vi "Binding Machine.vi"() -> ()   [LabVIEW 2014]
uses:
  Master/Master.lvclass
panel:
  in  "Enter":bool
  in  "stop":bool
  out "error out":errorcluster
  in  "error in":errorcluster
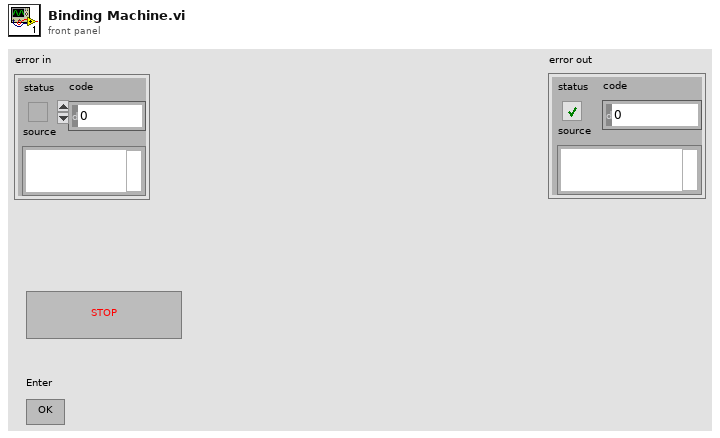
[diagram p1: front panel]
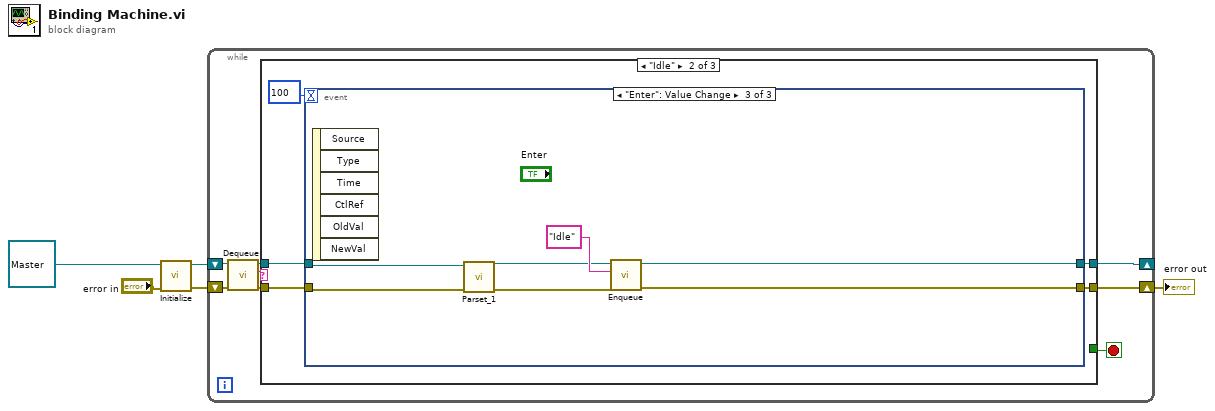
[diagram p0: block diagram]
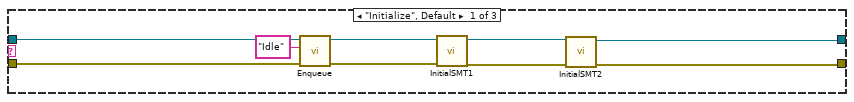
[diagram p2: hidden frame]
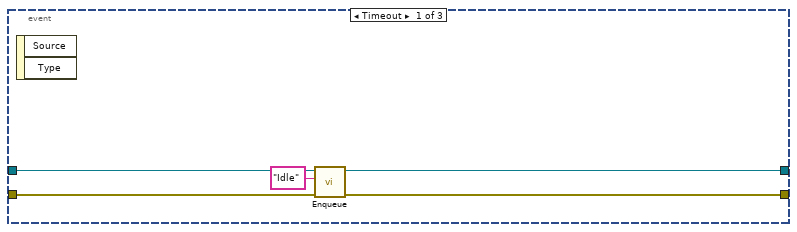
[diagram p3: hidden frame]
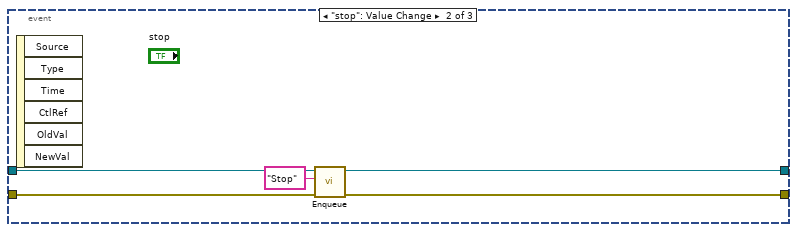
[diagram p4: hidden frame]
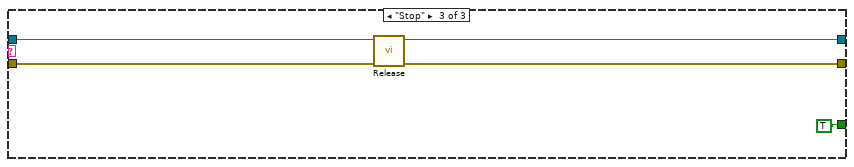
[diagram p5: hidden frame]
diagram:
  n1 = call-dynamic "Initialize.vi"("error in (no error)"="error in", "Master in"=refnum<class "Master.lvclass"> refnum ("Master.lvclass")) -> ("error out"=w2:errorcluster, "Master out"=w3:refnum<class "Master.lvclass">)  [unwired: 8 in]
  n2 = while {
    shift-right: [w9] -> _
    shift-left: w3 -> [w13]
    shift-right: [w7] -> w5
    shift-left: w2 -> [w12]
    stop <- w6 stop-if-true
    n3 = call-dynamic "Dequeue.vi"("error in (no error)"=w12, "Master in"=w13) -> ("error out"=w8:errorcluster, "State"=w11:string, "Master out"=w10:refnum<class "Master.lvclass">)  [unwired: 7 in]
    n4 = case shown="\"Idle\"" w11 {
      tunnel: w10 -> [w20 w26 w48]
      tunnel: [w16 w23 w46] -> w9
      tunnel: w8 -> [w22 w25 w47]
      tunnel: [w14 w24 w45] -> w7
      tunnel: [_ _ TRUE] -> w6
      frame "Initialize", Default {
        n5 = call-dynamic "Enqueue.vi"("error in (no error)"=w22, "State"="Idle", "Master in"=w20) -> ("error out"=w18:errorcluster, "Master out"=w19:refnum<class "Master.lvclass">)  [unwired: 7 in]
        n6 = call-dynamic "InitialSMT1.vi"("error in (no error)"=w18, "Programing Logic in"=w19) -> ("error out"=w15:errorcluster, "Programing Logic out"=w17:refnum<class "Master.lvclass">)  [unwired: 8 in]
        n7 = call-dynamic "InitialSMT2.vi"("error in (no error)"=w15, "Programing Logic in"=w17) -> ("error out"=w14:errorcluster, "Programing Logic out"=w16:refnum<class "Master.lvclass">)  [unwired: 8 in]
      }
      frame "Idle" {
        n8 = event shown="[2] \"Enter\": Value Change" {
          selector: _ -> [_ _ _]
          dyn-events: _ -> [_ _ _]
          timeout: 100 -> [_ _ _]
          tunnel: w26 -> [w32 w37 w43]
          tunnel: w25 -> [w31 w36 w42]
          tunnel: [w30 w35 w39] -> w24
          tunnel: [w29 w34 w38] -> w23
          event Timeout {
            n9 = event-data() -> ()  [unwired: 1 in, 2 out]
            n10 = call-dynamic "Enqueue.vi"("error in (no error)"=w31, "State"="Idle", "Master in"=w32) -> ("error out"=w30:errorcluster, "Master out"=w29:refnum<class "Master.lvclass">)  [unwired: 7 in]
          }
          event "stop": Value Change {
            n11 = event-data() -> ()  [unwired: 1 in, 6 out]
            n12 = call-dynamic "Enqueue.vi"("error in (no error)"=w36, "State"="Stop", "Master in"=w37) -> ("error out"=w35:errorcluster, "Master out"=w34:refnum<class "Master.lvclass">)  [unwired: 7 in]
          }
          event "Enter": Value Change {
            n13 = event-data() -> ()  [unwired: 1 in, 6 out]
            n14 = call-dynamic "Parset_1.vi"("error in (no error)"=w42, "Programing Logic in"=w43) -> ("error out"=w40:errorcluster, "Programing Logic out"=w41:refnum<class "Master.lvclass">)  [unwired: 8 in]
            n15 = call-dynamic "Enqueue.vi"("error in (no error)"=w40, "State"="Idle", "Master in"=w41) -> ("error out"=w39:errorcluster, "Master out"=w38:refnum<class "Master.lvclass">)  [unwired: 7 in]
          }
        }
      }
      frame "Stop" {
        n16 = call-dynamic "Release.vi"("error in (no error)"=w47, "Master in"=w48) -> ("error out"=w45:errorcluster, "Master out"=w46:refnum<class "Master.lvclass">)  [unwired: 8 in]
      }
    }
  }
  "error out" <- w5
